vi "AddKeyboardState.vi"(8 "error in (no error)":errorcluster, 10 "Keyboard State":T1, 11 "Input in":refnum<class "Input.lvclass">) -> (0 "error out":errorcluster, 3 "Input out":refnum<class "Input.lvclass">)   [LabVIEW 2015]
uses:
  Input.lvclass
  Keyboard State.ctl
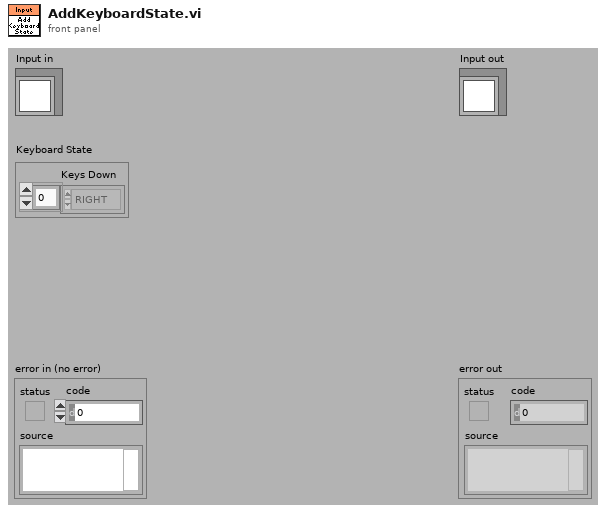
[diagram p1: front panel]
types:
  T1 = typedef "Input.lvclass/Keyboard State.ctl" = cluster{"Keys Down":enum16{"0", "1", "2", "3", "4", "5", "6", "7", "8", "9", "A", "B", "C", "D", "E", "F", "G", "H", "I", "J", "K", "L", "M", "N", "O", "P", "Q", "R", "S", "T", "U", "V", "W", "X", "Y", "Z", "F1", "F2", "F3", "F4", "F5", "F6", "F7", "F8", "F9", "F10", "F11", "F12", "F13", "F14", "F15", "ADD", "BACK", "BACKSLASH", "CAPITAL", "COMMA", "DECIMAL", "DELETE", "DIVIDE", "DOWN", "END", "EQUALS", "ESCAPE", "GRAVE (`)", "HOME", "INSERT", "LBRACKET", "LCONTROL", "LEFT", "L ALT", "LSHIFT", "LWIN", "MINUS", "MULTIPLY", "NEXT", "NUMLOCK", "NUMPAD_0", "NUMPAD_1", "NUMPAD_2", "NUMPAD_3", "NUMPAD_4", "NUMPAD_5", "NUMPAD_6", "NUMPAD_7", "NUMPAD_8", "NUMPAD_9", "PAUSE", "PERIOD", "PRIOR (PG UP)", "RBRACKET", "RCONTROL", "RETURN", "RIGHT", "R ALT", "RSHIFT", "RWIN", "SCROLL", "SEMICOLON", "SLASH", "SPACE", "SUBTRACT", "TAB", "UP", "ENTER (num pad)", "' (quote)"}[]}
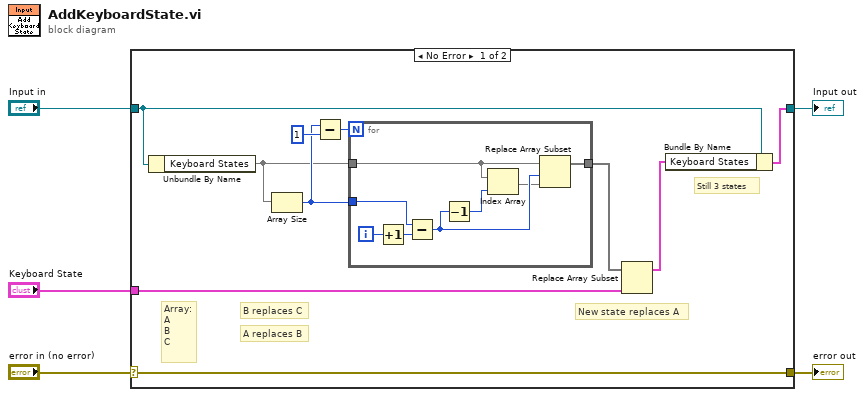
[diagram p0: block diagram]
diagram:
  n1 = case shown="No Error" "error in (no error)" {
    selector: "error in (no error)" -> [w15 w25]
    tunnel: [w15 w25] -> w4
    tunnel: [w7 w24] -> w2
    tunnel: "Input in" -> [w8 w24]
    tunnel: "Keyboard State" -> [w6 _]
    frame No Error {
      # "Still 3 states"
      # "New state replaces A"
      # "A replaces B"
      # "B replaces C"
      # "Array:\nA\nB\nC"
      n2 = Unbundle By Name(w8) -> ("Keyboard States"=w9)
      n3 = Array Size(array=w9) -> (size(s)=w10:i32)
      n4 = Subtract(x=w10, y=1 ("x")) -> (x-y=w11:i32)
      n5 = for {
        N: w11 -> [_]
        tunnel: w9 -> [w21]
        tunnel: w10 -> [w17]
        tunnel: [w16] -> w13
        i -> [w23]
        n6 = Increment(x=w23) -> (x+1=w22:i32)
        n7 = Subtract(x=w17, y=w22) -> (x-y=w20:i32)
        n8 = Decrement(x=w20) -> (x-1=w19:i32)
        n9 = Index Array(array=w21, index=w19) -> (element=w18)
        n10 = Replace Array Subset(array=w21, new element=w18, index=w20) -> (w16:void[])
      }
      n11 = Replace Array Subset(array=w13, new element=w6) -> (w14:T1[])  [unwired: 1 in]
      n12 = Bundle By Name(cluster=w8, "Keyboard States"=w14) -> (w7:cluster{})
    }
    frame Error {
    }
  }
  "error out" <- w4
  "Input out" <- w2
